vi "Untitled 1.vi"() -> ()   [LabVIEW 2018]
uses:
  #include/Global textParse.vi
  <instrlib>/RIGOL DS1000 Series/RIGOL DS1000 Series.lvlib
panel:
  in  "E-Stop":bool
  out "Vpass2":bool
  out "Vpass1":bool
  out "Vpass1 Measure":dbl
  out "Vpass2 Measure":dbl
  out "Vload":bool
  out "Vload Measure":dbl
  out "Vrip":bool
  out "Vrip Measure":dbl
  out "Vout":bool
  out "Vout Measure":dbl
  out "refnum out":refnum<file>
  in  "VISA Waveform Generator":refnum<visa-resource-name>
  in  "VISA Oscilloscope":refnum<visa-resource-name>
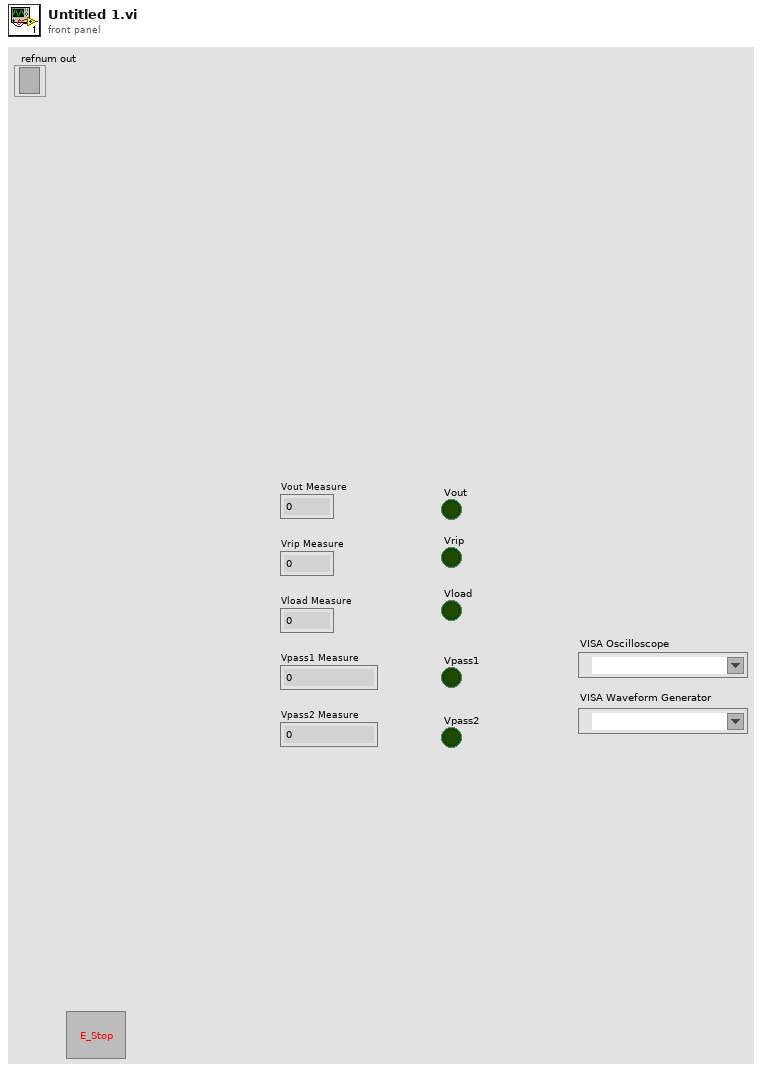
[diagram p1: front panel]
types:
  T1 = enum16{"scope", "Vout", "Vload", "Vpass", "end", ""}
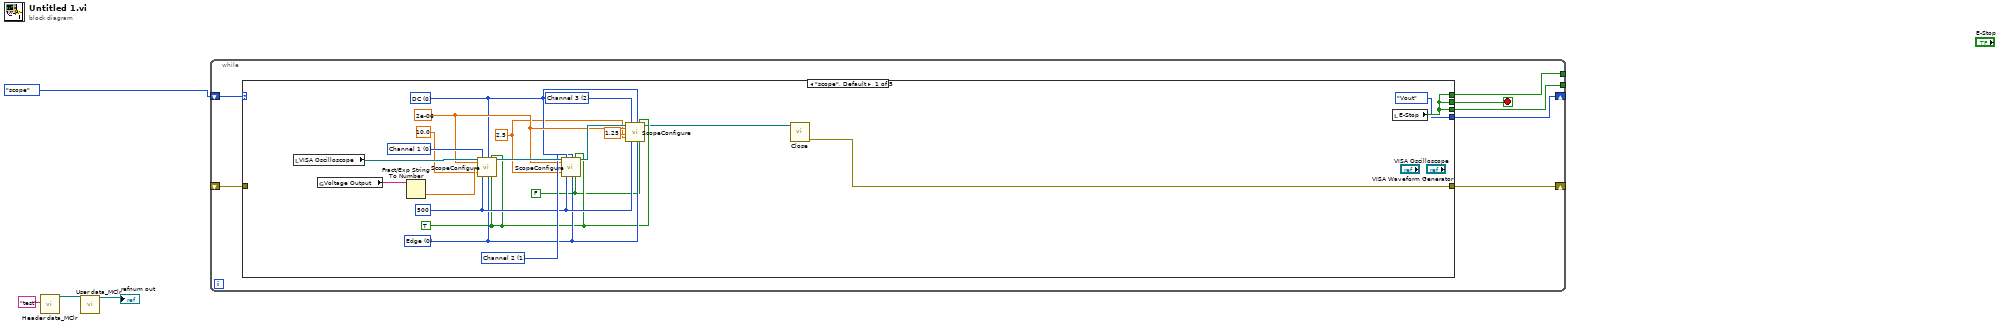
[diagram p0: block diagram]
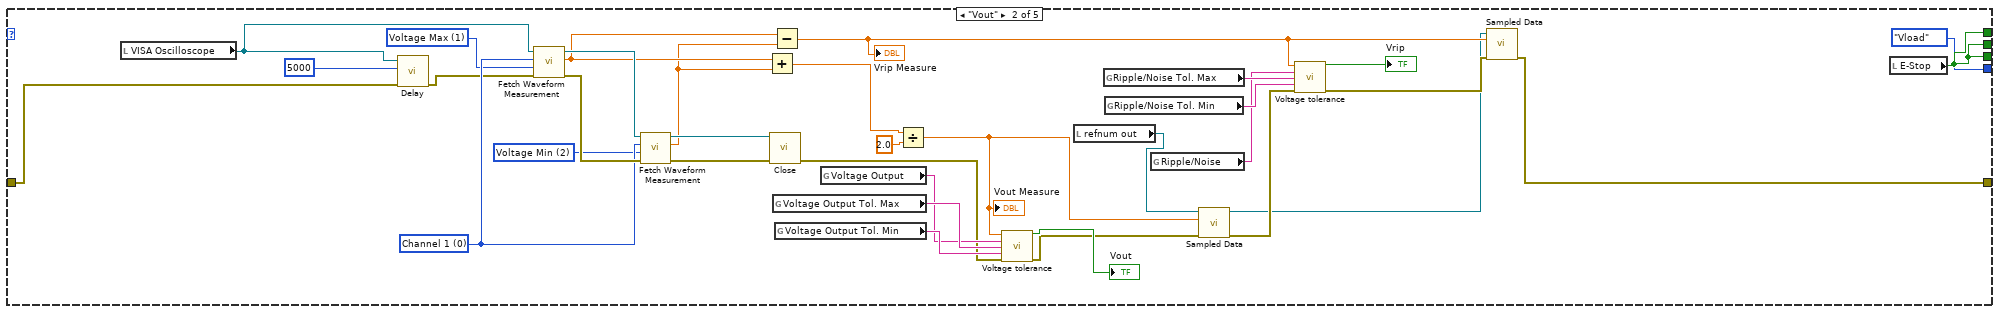
[diagram p2: hidden frame]
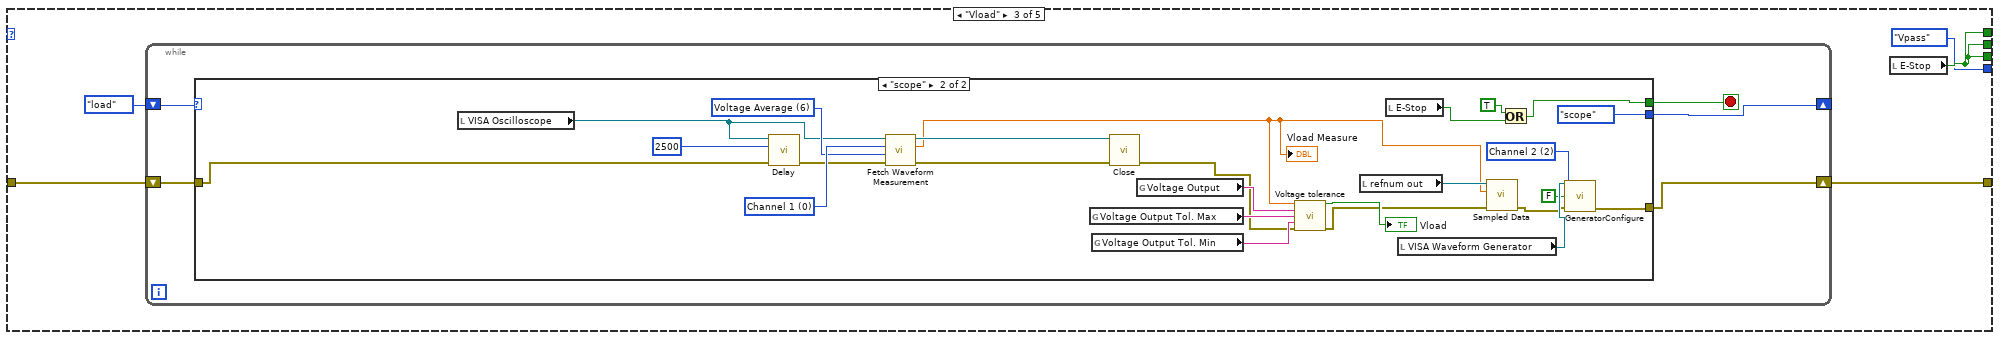
[diagram p3: hidden frame]
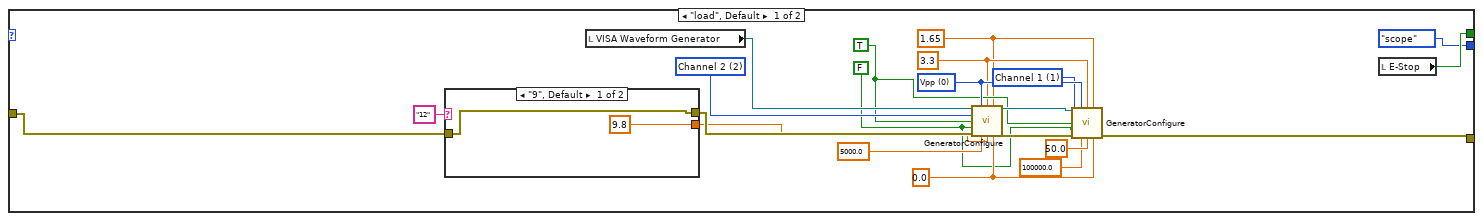
[diagram p4: hidden frame]
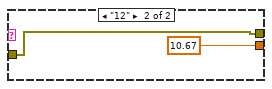
[diagram p5: hidden frame]
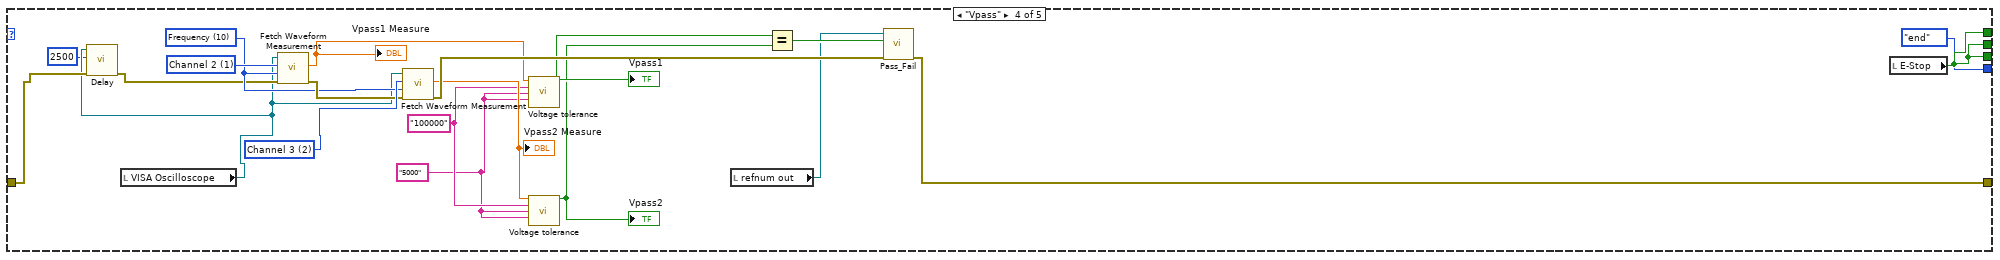
[diagram p6: hidden frame]
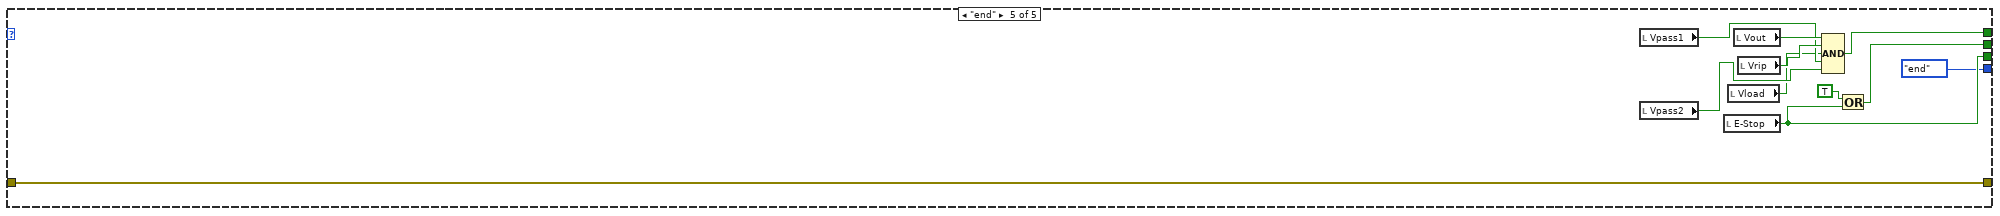
[diagram p7: hidden frame]
diagram:
  n1 = call "Header data_MClr.vi"("file name"="test") -> ("refnum out"=w3:refnum<file>)  [unwired: 17 in, 1 out]
  n2 = call "User data_MClr.vi"("refnum in"=w3) -> ("refnum out"=→"refnum out":refnum<file>)  [unwired: 7 in, 1 out]
  n3 = while {
    shift-right: [w5] -> _
    shift-left: T1."scope" -> [w11]
    shift-right: [w8] -> _
    shift-left: _ -> [w9]
    tunnel: [w7] -> _
    tunnel: [w6] -> _
    stop <- w10 stop-if-true
    n4 = case shown="\"scope\", Default" w11 {
      tunnel: [w19 w60 w68 w139 w148] -> w10
      tunnel: w9 -> [_ w35 w70 w130 w157]
      tunnel: [w16 w62 w69 w144 w157] -> w8
      tunnel: [w19 w60 w68 w139 w152] -> w7
      tunnel: [w19 w60 w68 w139 w150] -> w6
      tunnel: [T1."Vout" T1."Vload" T1."Vpass" T1."end" T1."end"] -> w5
      frame "scope", Default {
        w12 = FALSE
        w13 = 2.5
        w26 = u16 2 items=["Channel 1", "Channel 2", "Channel 3", "Channel 4"] ("Channel (0: Channel 1)")
        w27 = u16 1 items=["Channel 1", "Channel 2", "Channel 3", "Channel 4"] ("Channel (0: Channel 1)")
        w23 = u16 0 items=["Edge", "Pulse", "Video", "Pattern", "Duration"] ("Trigger Type (0: Edge)")
        w25 = 2e-06
        w22 = u16 0 items=["DC", "AC", "Ground"] ("Vertical Coupling (0: DC)")
        w30 = u16 0 items=["Channel 1", "Channel 2", "Channel 3", "Channel 4"] ("Channel (0: Channel 1)")
        w24 = 500 ("Attenuation")
        w20 = TRUE
        n5 = local read "VISA Oscilloscope"() -> (w31:refnum<visa-resource-name>)
        n6 = global read "Global textParse.vi" "Voltage Output"() -> (w32:string)
        n7 = Fract/Exp String To Number(string=w32) -> (number=w21:dbl)  [unwired: 3 in, 1 out]
        n8 = call "ScopeConfigure.vi"("VISA resource name"=w31, "scaleTime"=w25, "triggerVoltage"=w21, "scaleVoltage"=10.0, "Channel (0: Channel 1)"=w30, "Attenuation"=w24, "Vertical Coupling (0: DC)"=w22, "Trigger Type (0: Edge)"=w23, "BW Selector"=w20, "F Selector"=w20) -> ("VISA resource name out"=w29:refnum<visa-resource-name>)  [unwired: 9 in]
        n9 = call "ScopeConfigure.vi"("VISA resource name"=w29, "scaleTime"=w25, "scaleVoltage"=w13, "Channel (0: Channel 1)"=w27, "Attenuation"=w24, "Vertical Coupling (0: DC)"=w22, "Trigger Type (0: Edge)"=w23, "BW Selector"=w20, "F Selector"=w12) -> ("VISA resource name out"=w28:refnum<visa-resource-name>)  [unwired: 10 in]
        n10 = call "ScopeConfigure.vi"("VISA resource name"=w28, "scaleTime"=w25, "triggerVoltage"=1.25 ("Trigger Level"), "scaleVoltage"=w13, "Channel (0: Channel 1)"=w26, "Attenuation"=w24, "Vertical Coupling (0: DC)"=w22, "Trigger Type (0: Edge)"=w23, "BW Selector"=w20, "F Selector"=w12) -> ("VISA resource name out"=w15:refnum<visa-resource-name>)  [unwired: 9 in]
        n11 = call <instrlib>:"Close.vi"("VISA resource name"=w15) -> ("error out"=w16:errorcluster)  [unwired: 10 in]
        n12 = local read "E-Stop"() -> (w19:bool)
      }
      frame "Vout" {
        w51 = u16 2 items=["Voltage Vpp", "Voltage Max", "Voltage Min", "Amplitude", "Voltage TOP", "Voltage Base", "Voltage Average", "Voltage RMS", "Overshoot", "Preshoot", "Frequency", "Rise Time", "Fall Time", "Period", "Positive Width", "Negative Width", "Positive Duty", "Negative Duty"] ("Measurement Function (0: Voltage Vpp)")
        w52 = u16 1 items=["Voltage Vpp", "Voltage Max", "Voltage Min", "Amplitude", "Voltage TOP", "Voltage Base", "Voltage Average", "Voltage RMS", "Overshoot", "Preshoot", "Frequency", "Rise Time", "Fall Time", "Period", "Positive Width", "Negative Width", "Positive Duty", "Negative Duty"] ("Measurement Function (0: Voltage Vpp)")
        w53 = u16 0 items=["Channel 1", "Channel 2", "Channel 3", "Channel 4"] ("Source (0: Channel 1)")
        n13 = local read "VISA Oscilloscope"() -> (w34:refnum<visa-resource-name>)
        n14 = call <instrlib>:"Delay.vi"("error in (no error)"=w35, "Delay (ms)"=u32 5000, "VISA resource name"=w34) -> ("error out"=w36:errorcluster)  [unwired: 7 in, 1 out]
        n15 = call <instrlib>:"Fetch Waveform Measurement.vi"("error in (no error)"=w36, "Measurement Function (0: Voltage Vpp)"=w52, "Source (0: Channel 1)"=w53, "VISA resource name"=w34) -> ("error out"=w54:errorcluster, "Measured Value"=w39:dbl, "VISA resource name out"=w55:refnum<visa-resource-name>)  [unwired: 5 in]
        n16 = call <instrlib>:"Fetch Waveform Measurement.vi"("error in (no error)"=w54, "Measurement Function (0: Voltage Vpp)"=w51, "Source (0: Channel 1)"=w53, "VISA resource name"=w55) -> ("error out"=w56:errorcluster, "Measured Value"=w38:dbl, "VISA resource name out"=w57:refnum<visa-resource-name>)  [unwired: 5 in]
        n17 = Add(x=w39, y=w38) -> (x+y=w50:dbl)
        n18 = call <instrlib>:"Close.vi"("error in (no error)"=w56, "VISA resource name"=w57) -> ("error out"=w37:errorcluster)  [unwired: 9 in]
        n19 = Subtract(x=w39, y=w38) -> (x-y=w63:dbl)
        "Vrip Measure" <- w63
        n20 = global read "Global textParse.vi" "Voltage Output Tol. Max"() -> (w46:string)
        n21 = global read "Global textParse.vi" "Voltage Output Tol. Min"() -> (w47:string)
        n22 = global read "Global textParse.vi" "Voltage Output"() -> (w45:string)
        n23 = Divide(x=w50, y=2.0) -> (x/y=w40:dbl)
        "Vout Measure" <- w40
        n24 = call "Voltage tolerance.vi"("Data Sample"=w40, "Spec Output"=w45, "Upper"=w46, "Lower"=w47, "error in (no error)"=w37) -> ("Boolean"=→"Vout":bool, "error out"=w44:errorcluster)  [unwired: 9 in]
        n25 = local read "refnum out"() -> (w41:refnum<file>)
        n26 = global read "Global textParse.vi" "Ripple/Noise Tol. Max"() -> (w66:string)
        n27 = global read "Global textParse.vi" "Ripple/Noise Tol. Min"() -> (w65:string)
        n28 = global read "Global textParse.vi" "Ripple/Noise"() -> (w59:string)
        n29 = call "Sampled Data.vi"("Error In"=w44, "Data Sample"=w40, "refnum in"=w41) -> ("error out"=w43:errorcluster, "refnum out"=w42:refnum<file>)  [unwired: 7 in]
        n30 = call "Voltage tolerance.vi"("Data Sample"=w63, "Spec Output"=w59, "Upper"=w66, "Lower"=w65, "error in (no error)"=w43) -> ("Boolean"=→"Vrip":bool, "error out"=w64:errorcluster)  [unwired: 9 in]
        n31 = call "Sampled Data.vi"("Error In"=w64, "Data Sample"=w63, "refnum in"=w42) -> ("error out"=w62:errorcluster)  [unwired: 7 in, 1 out]
        n32 = local read "E-Stop"() -> (w60:bool)
      }
      frame "Vload" {
        n33 = while {
          shift-right: [w72] -> _
          shift-left: enum16{"load", "scope"}."load" -> [w76]
          shift-right: [w73] -> w69
          shift-left: w70 -> [w74]
          stop <- w75 stop-if-true
          n34 = case shown="\"scope\"" w76 {
            tunnel: [w97 w113] -> w75
            tunnel: w74 -> [w96 w111]
            tunnel: [w87 w102] -> w73
            tunnel: [enum16{"load", "scope"}."scope" enum16{"load", "scope"}."scope"] -> w72
            frame "load", Default {
              w82 = 1 items=["Channel 1"=1, "Channel 2"=2] ("Output Channel (1: Channel 1)")
              w86 = 0 items=["Vpp", "Vrms", "dBm"] ("Amplitude Unit (0: Vpp)")
              w85 = 0.0 ("Phase (0 Degree)")
              w93 = 2 items=["Channel 1"=1, "Channel 2"=2] ("Output Channel (1: Channel 1)")
              w80 = FALSE ("Enable Output 1")
              w78 = 1.65
              w79 = 3.3
              w81 = TRUE
              n35 = case shown="\"9\", Default" "12" {
                tunnel: [9.8 10.67] -> w91
                tunnel: w96 -> [w98 w100]
                tunnel: [w98 w100] -> w94
                frame "9", Default {
                }
                frame "12" {
                }
              }
              n36 = local read "VISA Waveform Generator"() -> (w92:refnum<visa-resource-name>)
              n37 = call "GeneratorConfigure.vi"("VISA resource name"=w92, "Amplitude Unit (0: Vpp)"=w86, "Amplitude (5 Vpp)"=w79, "Offset (0)"=w78, "Output Channel (1: Channel 1)"=w93, "Enable Output (T: Enable)"=w81, "Enable Align (F: Disable)"=w80, "error in (no error)"=w94, "Frequency (1000 Hz)"=5000.0, "Duty Cycle (50 %)"=w91, "Phase (0 Degree)"=w85) -> ("VISA resource name out"=w89:refnum<visa-resource-name>, "error out"=w88:errorcluster)  [unwired: 3 in]
              n38 = call "GeneratorConfigure.vi"("VISA resource name"=w89, "Amplitude Unit (0: Vpp)"=w86, "Amplitude (5 Vpp)"=w79, "Offset (0)"=w78, "Output Channel (1: Channel 1)"=w82, "Enable Output (T: Enable)"=w81, "Enable Align (F: Disable)"=w80, "error in (no error)"=w88, "Frequency (1000 Hz)"=100000.0, "Duty Cycle (50 %)"=50.0, "Phase (0 Degree)"=w85) -> ("error out"=w87:errorcluster)  [unwired: 3 in, 1 out]
              n39 = local read "E-Stop"() -> (w97:bool)
            }
            frame "scope" {
              w105 = 2 items=["Channel 1"=1, "Channel 2"=2] ("Output Channel (1: Channel 1)")
              w123 = u16 6 items=["Voltage Vpp", "Voltage Max", "Voltage Min", "Amplitude", "Voltage TOP", "Voltage Base", "Voltage Average", "Voltage RMS", "Overshoot", "Preshoot", "Frequency", "Rise Time", "Fall Time", "Period", "Positive Width", "Negative Width", "Positive Duty", "Negative Duty"] ("Measurement Function (0: Voltage Vpp)")
              w125 = u16 0 items=["Channel 1", "Channel 2", "Channel 3", "Channel 4"] ("Channel (0: Channel 1)")
              n40 = local read "VISA Oscilloscope"() -> (w109:refnum<visa-resource-name>)
              n41 = call <instrlib>:"Delay.vi"("error in (no error)"=w111, "Delay (ms)"=u32 2500, "VISA resource name"=w109) -> ("error out"=w110:errorcluster)  [unwired: 7 in, 1 out]
              n42 = call <instrlib>:"Fetch Waveform Measurement.vi"("error in (no error)"=w110, "Measurement Function (0: Voltage Vpp)"=w123, "Source (0: Channel 1)"=w125, "VISA resource name"=w109) -> ("error out"=w126:errorcluster, "Measured Value"=w107:dbl, "VISA resource name out"=w124:refnum<visa-resource-name>)  [unwired: 5 in]
              "Vload Measure" <- w107
              n43 = global read "Global textParse.vi" "Voltage Output Tol. Max"() -> (w121:string)
              n44 = global read "Global textParse.vi" "Voltage Output Tol. Min"() -> (w120:string)
              n45 = call <instrlib>:"Close.vi"("error in (no error)"=w126, "VISA resource name"=w124) -> ("error out"=w119:errorcluster)  [unwired: 9 in]
              n46 = global read "Global textParse.vi" "Voltage Output"() -> (w122:string)
              n47 = call "Voltage tolerance.vi"("Data Sample"=w107, "Spec Output"=w122, "Upper"=w121, "Lower"=w120, "error in (no error)"=w119) -> ("Boolean"=→"Vload":bool, "error out"=w116:errorcluster)  [unwired: 9 in]
              n48 = local read "refnum out"() -> (w117:refnum<file>)
              n49 = local read "E-Stop"() -> (w114:bool)
              n50 = local read "VISA Waveform Generator"() -> (w106:refnum<visa-resource-name>)
              n51 = call "Sampled Data.vi"("Error In"=w116, "Data Sample"=w107, "refnum in"=w117) -> ("error out"=w103:errorcluster)  [unwired: 7 in, 1 out]
              n52 = Or(x=TRUE, y=w114) -> (x .or. y?=w113:bool)
              n53 = call "GeneratorConfigure.vi"("VISA resource name"=w106, "Output Channel (1: Channel 1)"=w105, "Enable Output (T: Enable)"=FALSE, "error in (no error)"=w103) -> ("error out"=w102:errorcluster)  [unwired: 10 in, 1 out]
            }
          }
        }
        n54 = local read "E-Stop"() -> (w68:bool)
      }
      frame "Vpass" {
        w131 = "5000"
        w132 = "100000"
        w140 = u16 10 items=["Voltage Vpp", "Voltage Max", "Voltage Min", "Amplitude", "Voltage TOP", "Voltage Base", "Voltage Average", "Voltage RMS", "Overshoot", "Preshoot", "Frequency", "Rise Time", "Fall Time", "Period", "Positive Width", "Negative Width", "Positive Duty", "Negative Duty"] ("Measurement Function (0: Voltage Vpp)")
        w145 = u16 2 items=["Channel 1", "Channel 2", "Channel 3", "Channel 4"] ("Channel (0: Channel 1)")
        w146 = u16 1 items=["Channel 1", "Channel 2", "Channel 3", "Channel 4"] ("Channel (0: Channel 1)")
        n55 = local read "VISA Oscilloscope"() -> (w128:refnum<visa-resource-name>)
        n56 = call <instrlib>:"Delay.vi"("error in (no error)"=w130, "Delay (ms)"=u32 2500, "VISA resource name"=w128) -> ("error out"=w129:errorcluster)  [unwired: 7 in, 1 out]
        n57 = call <instrlib>:"Fetch Waveform Measurement.vi"("error in (no error)"=w129, "Measurement Function (0: Voltage Vpp)"=w140, "Source (0: Channel 1)"=w146, "VISA resource name"=w128) -> ("error out"=w142:errorcluster, "Measured Value"=w138:dbl)  [unwired: 5 in, 1 out]
        "Vpass1 Measure" <- w138
        n58 = call <instrlib>:"Fetch Waveform Measurement.vi"("error in (no error)"=w142, "Measurement Function (0: Voltage Vpp)"=w140, "Source (0: Channel 1)"=w145, "VISA resource name"=w128) -> ("error out"=w141:errorcluster, "Measured Value"=w137:dbl)  [unwired: 5 in, 1 out]
        "Vpass2 Measure" <- w137
        n59 = call "Voltage tolerance.vi"("Data Sample"=w138, "Spec Output"=w132, "Upper"=w131, "Lower"=w131) -> ("Boolean"=w136:bool)  [unwired: 10 in, 1 out]
        "Vpass1" <- w136
        n60 = call "Voltage tolerance.vi"("Data Sample"=w137, "Spec Output"=w132, "Upper"=w131, "Lower"=w131) -> ("Boolean"=w135:bool)  [unwired: 10 in, 1 out]
        "Vpass2" <- w135
        n61 = local read "refnum out"() -> (w133:refnum<file>)
        n62 = Equal?(x=w136, y=w135) -> (x = y?=w143:bool)
        n63 = call "Pass_Fail.vi"("error in (no error)"=w141, "OK"=w143, "Byte Stream File in"=w133) -> ("error out"=w144:errorcluster)  [unwired: 7 in, 1 out]
        n64 = local read "E-Stop"() -> (w139:bool)
      }
      frame "end" {
        n65 = local read "Vpass1"() -> (w154:bool)
        n66 = local read "Vpass2"() -> (w153:bool)
        n67 = local read "E-Stop"() -> (w150:bool)
        n68 = local read "Vload"() -> (w151:bool)
        n69 = local read "Vout"() -> (w156:bool)
        n70 = local read "Vrip"() -> (w155:bool)
        n71 = Compound Arithmetic op=AND(w156, w155, w151, w154, w153) -> (w152:bool)
        n72 = Or(x=TRUE, y=w150) -> (x .or. y?=w148:bool)
      }
    }
  }
